vi "niFpgaFFTPermutationLargeTemp.vi"(6 "perm switch":bool, 9 "stage switch":bool, 11 "bf data in":T1 {"x_r" format="%.16g"; "x_i" format="%.16g"; "y_r" format="%.16g"; "y_i" format="%.16g"}) -> (3 "bf data out":T1 {"x_r" format="%.16g"; "x_i" format="%.16g"; "y_r" format="%.16g"; "y_i" format="%.16g"})   [LabVIEW 2017]
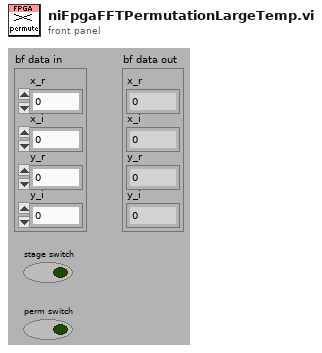
[diagram p1: front panel]
types:
  T1 = cluster{"x_r":fxp<+/-,16,1>, "x_i ":fxp<+/-,16,1>, "y_r ":fxp<+/-,16,1>, "y_i ":fxp<+/-,16,1>}
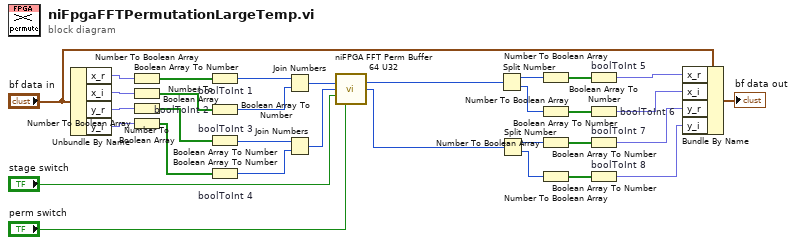
[diagram p0: block diagram]
diagram:
  n1 = Unbundle By Name("bf data in") -> ("x_r"=w26:fxp<+/-,16,1>, "x_i"=w25:fxp<+/-,16,1>, "y_r"=w24:fxp<+/-,16,1>, "y_i"=w23:fxp<+/-,16,1>)
  n2 = Number To Boolean Array(number=w26) -> (Boolean array=w9:bool[])
  n3 = Number To Boolean Array(number=w25) -> (Boolean array=w8:bool[])
  n4 = Number To Boolean Array(number=w24) -> (Boolean array=w7:bool[])
  n5 = Number To Boolean Array(number=w23) -> (Boolean array=w6:bool[])
  n6 = Boolean Array To Number "boolToInt 1"(Boolean array=w9) -> (number=w3:u16)
  n7 = Boolean Array To Number "boolToInt 2"(Boolean array=w8) -> (number=w2:u16)
  n8 = Boolean Array To Number "boolToInt 3"(Boolean array=w7) -> (number=w4:u16)
  n9 = Boolean Array To Number "boolToInt 4"(Boolean array=w6) -> (number=w5:u16)
  n10 = Join Numbers(hi=w3, lo=w2) -> ((hi.lo)=w22:u32)
  n11 = Join Numbers(hi=w4, lo=w5) -> ((hi.lo)=w29:u32)
  n12 = call <vilib>:"niFPGA FFT Perm Buffer 64 U32.vi"("x in"=w22, "y in"=w29, "stage switch"="stage switch", "Switch"="perm switch") -> ("x out"=w28:u32, "y out"=w27:u32)  [unwired: 10 out]
  n13 = Split Number(x=w28) -> (hi(x)=w31:u16, lo(x)=w32:u16)
  n14 = Split Number(x=w27) -> (hi(x)=w1:u16, lo(x)=w30:u16)
  n15 = Number To Boolean Array(number=w31) -> (Boolean array=w17:bool[])
  n16 = Number To Boolean Array(number=w32) -> (Boolean array=w16:bool[])
  n17 = Number To Boolean Array(number=w1) -> (Boolean array=w15:bool[])
  n18 = Number To Boolean Array(number=w30) -> (Boolean array=w14:bool[])
  n19 = Boolean Array To Number "boolToInt 5"(Boolean array=w17) -> (number=w12:fxp<+/-,16,1>)
  n20 = Boolean Array To Number "boolToInt 6"(Boolean array=w16) -> (number=w11:fxp<+/-,16,1>)
  n21 = Boolean Array To Number "boolToInt 7"(Boolean array=w15) -> (number=w10:fxp<+/-,16,1>)
  n22 = Boolean Array To Number "boolToInt 8"(Boolean array=w14) -> (number=w13:fxp<+/-,16,1>)
  n23 = Bundle By Name(cluster="bf data in", "x_r"=w12, "x_i"=w11, "y_r"=w10, "y_i"=w13) -> (→"bf data out":T1)
